vi "Configure Digital Channel.vi"(0 "VISA resource name":refnum<visa-resource-name>, 1 "Enable Channel (T: Enable)":bool=TRUE, 5 "Channel Name (0: DIG 0)":u16(ring) items=["DIG 0", "DIG 1", "DIG 2", "DIG 3", "DIG 4", "DIG 5", "DIG 6", "DIG 7", "DIG 8", "DIG 9", "DIG 10", "DIG 11", "DIG 12", "DIG 13", "DIG 14", "DIG 15"], 7 "Threshold (0: TTL)":u16(ring) items=["TTL", "CMOS", "ECL", "User Defined"], 9 "Threshold Value (0.0)":dbl, 11 "error in (no error)":errorcluster, 12 "Size (1:  Medium)":u16(ring)=1 items=["Small", "Medium", "Large"]) -> (4 "VISA resource name out":refnum<visa-resource-name>, 15 "error out":errorcluster)   [LabVIEW 2017, in "Agilent 6000 Series.lvlib"]
doc: "This VI configures the common properties of the oscilloscope's digital channel subsystem for a particular digital channel. These properties are the size, threshold, threshold value and channel enabled.\n\n<B>NOTE:</B>\n\nThis VI is only supported by MSO models; running this VI with a DSO model might throw an error."
uses:
  <instrlib>/Agilent 6000 Series/Agilent 6000 Series.lvlib
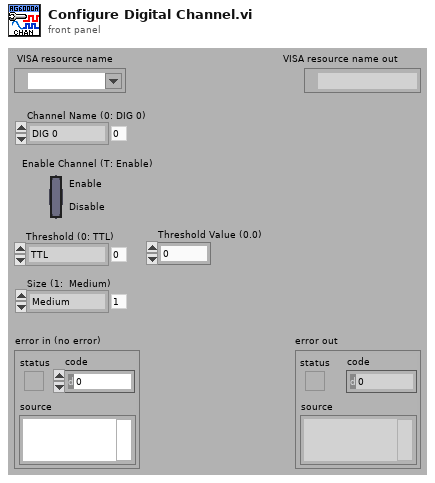
[diagram p1: front panel]
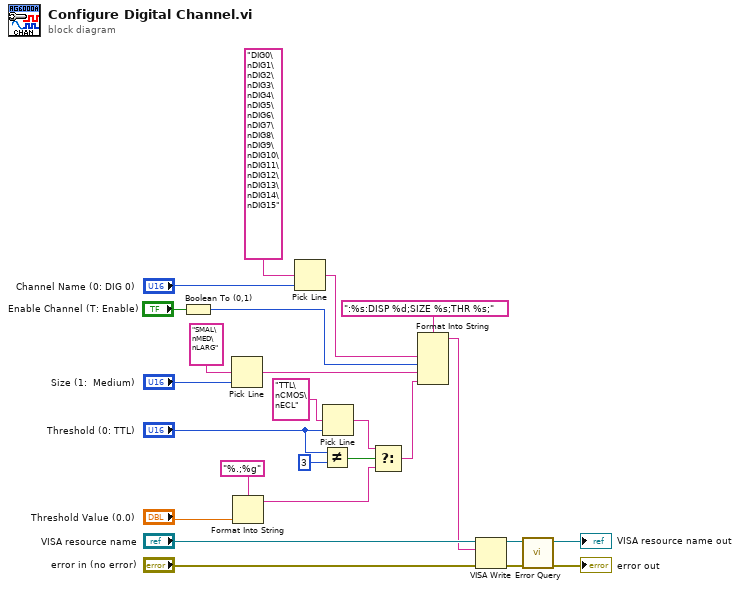
[diagram p0: block diagram]
diagram:
  n1 = Boolean To (0,1)(Boolean="Enable Channel (T: Enable)") -> (0, 1=w3:i16)
  n2 = Pick Line(multi-line string="SMAL\nMED\nLARG", line index="Size (1:  Medium)") -> (output string=w2:string)  [unwired: 1 in]
  n3 = Format Into String(format string="%.;%g", "Threshold Value (0.0)") -> (resulting string=w6:string)  [unwired: 2 in, 1 out]
  n4 = Pick Line(multi-line string="DIG0\nDIG1\nDIG2\nDIG3\nDIG4\nDIG5\nDIG6\nDIG7\nDIG8\nDIG9\nDIG10\nDIG11\nDIG12\nDIG13\nDIG14\nDIG15", line index="Channel Name (0: DIG 0)") -> (output string=w14:string)  [unwired: 1 in]
  n5 = Not Equal?(x="Threshold (0: TTL)", y=u16 3) -> (x != y?=w10:bool)
  n6 = Pick Line(multi-line string="TTL\nCMOS\nECL", line index="Threshold (0: TTL)") -> (output string=w9:string)  [unwired: 1 in]
  n7 = Select(t=w9, s=w10, f=w6) -> (s? t:f=w1:string)
  n8 = Format Into String(format string=":%s:DISP %d;SIZE %s;THR %s;", w14, w3, w2, w1) -> (resulting string=w5:string)  [unwired: 2 in, 1 out]
  n9 = VISA Write(VISA resource name="VISA resource name", write buffer=w5, error in (no error)="error in (no error)") -> (VISA resource name out=w21:refnum<visa-resource-name>, error out=w20:errorcluster)  [unwired: 1 out]
  n10 = call <instrlib>:"Error Query.vi"("error in (no error)"=w20, "VISA resource name"=w21) -> ("error out"=→"error out":errorcluster, "VISA resource name out"=→"VISA resource name out":refnum<visa-resource-name>)  [unwired: 6 in, 2 out]
